vi "FGV Ausgang schalten.vi"(6 "Aktion":T1, 11 "Ausgang aktiv":bool) -> (3 "Ausgang aktiv":bool)   [LabVIEW 2020, in "Regler.lvlib"]
uses:
  Regler.lvlib
  Aktion Ausgang schalten.ctl
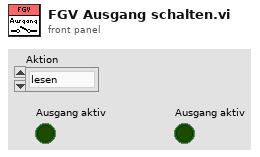
[diagram p1: front panel]
types:
  T1 = typedef "Regler.lvlib/Aktion Ausgang schalten.ctl" = enum16{"lesen", "schreiben"}
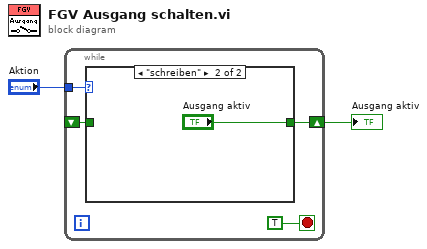
[diagram p0: block diagram]
diagram:
  n1 = while {
    tunnel: "Aktion" -> [w5]
    shift-right: [w4] -> w1
    shift-left: _ -> [w3]
    stop <- TRUE stop-if-true
    n2 = case shown="\"schreiben\"" w5 {
      tunnel: [w7 "Ausgang aktiv"] -> w4
      tunnel: w3 -> [w7 _]
      frame "lesen", Default {
      }
      frame "schreiben" {
      }
    }
  }
  "Ausgang aktiv" <- w1
